vi "leds_2_bit_array.vi"(11 "LEDs":u32[](array[numeric])) -> (3 "Bit Array":u8[](array[numeric]))   [LabVIEW 2013]
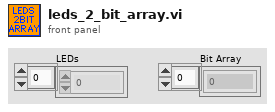
[diagram p1: front panel]
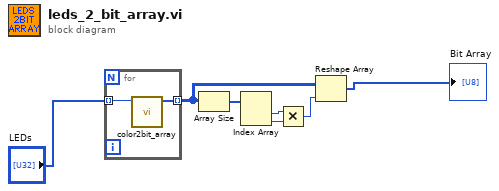
[diagram p0: block diagram]
diagram:
  n1 = for {
    tunnel: "LEDs" -> [w9] mode=indexing
    tunnel: [w8] -> w3 mode=indexing
    n2 = call "color2bit_array.vi"("Input Color"=w9) -> ("Bit Array"=w8:u8[])  [unwired: 10 in]
  }
  n3 = Array Size(array=w3) -> (size(s)=w4:i32[])
  n4 = Index Array(array=w4) -> (element #1=w6:i32, element #2=w5:i32)  [unwired: 2 in]
  n5 = Multiply(x=w6, y=w5) -> (x*y=w7:i32)
  n6 = Reshape Array(w3, w7) -> (→"Bit Array":u8[])
